vi "Quote and Escape JSON string.vi"(11 "Plain Text":string) -> (3 "<JSON>":string caption="JSON string (quoted and escaped)")   [LabVIEW 2019, in "JSONtext.lvlib"]
uses:
  JSONtext.lvlib
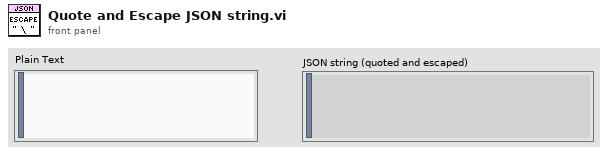
[diagram p1: front panel]
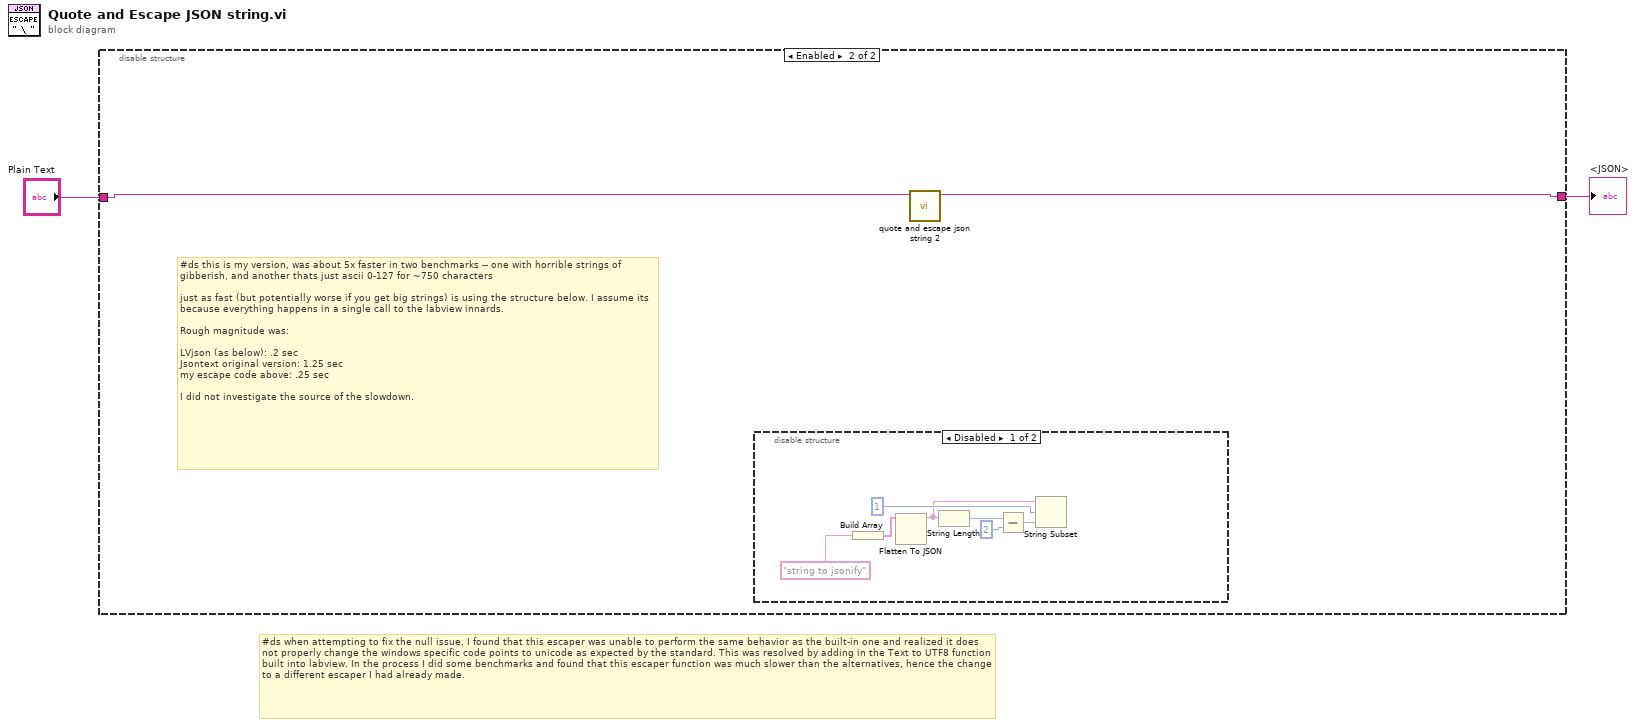
[diagram p0: block diagram]
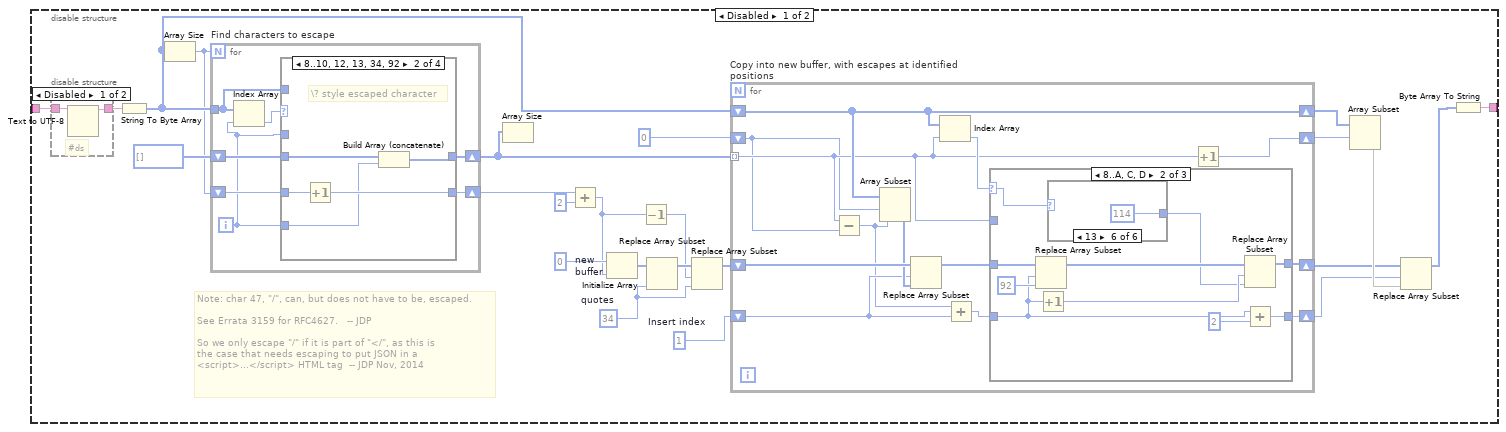
[diagram p2: hidden frame]
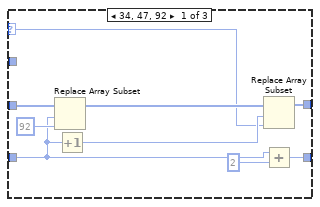
[diagram p4: hidden frame]
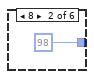
[diagram p6: hidden frame]
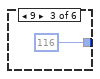
[diagram p7: hidden frame]
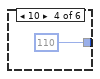
[diagram p8: hidden frame]
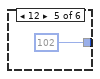
[diagram p9: hidden frame]
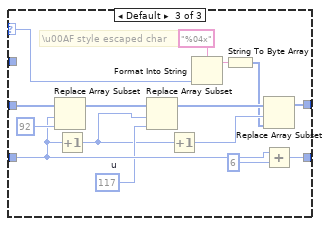
[diagram p10: hidden frame]
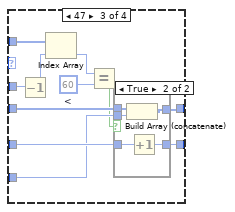
[diagram p12: hidden frame]
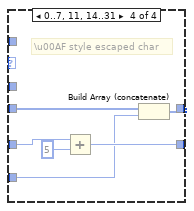
[diagram p14: hidden frame]
diagram:
  # "#ds when attempting to fix the null issue, I found that this escaper was unable to perform the same behavior as the built-in one and realized it does not properly change the windows specific code points to unicode as expected by the standard. This was resolved by adding in the Text to UTF8 function built into labview. In the process I did some benchmarks and found that this escaper function was much slower than the alternatives, hence the change to a different escaper I had already made."
  n1 = disable-structure shown="Enabled" {
    disable-tunnel: [w26 w120] -> w2
    disable-tunnel: "Plain Text" -> [w4 w121]
    frame Disabled {
      w7 = u8 34  # quotes
      w17 = 1  # Insert index
      # "Note: char 47, \"/\", can, but does not have to be, escaped.\n\nSee Errata 3159 for RFC4627.   -- JDP\n\nSo we only escape \"/\" if it is part of \"</\", as this is\nthe case that needs escaping to put JSON in a\n<script>...</script> HTML tag  -- JDP Nov, 2014"
      n2 = disable-structure shown="Disabled" {
        disable-tunnel: w4 -> [w28 w29]
        disable-tunnel: [w27 w29] -> w3
        frame Disabled {
          # "#ds"
          n3 = Text to UTF-8(11:w28) -> (3:w27:string)  [unwired: 2 in, 1 out]
        }
        frame Enabled {
        }
      }
      n4 = String To Byte Array(string=w3) -> (unsigned byte array=w21:u8[])
      n5 = Array Size(array=w21) -> (size(s)=w20:i32)
      n6 = for "Find characters to escape" {
        N: w20 -> [_]
        tunnel: w21 -> [w83]
        shift-right: [w87] -> w24
        shift-left: w20 -> [w88]
        shift-right: [w86] -> w22
        shift-left: i32[] [] -> [w85]
        i -> [w82]
        n7 = Index Array(array=w83, index=w82) -> (element=w84:u8)
        n8 = case shown="8..10, 12, 13, 34, 92" w84 {
          tunnel: w88 -> [w90 w95 w106 w116]
          tunnel: [w90 w94 w105 w119] -> w87
          tunnel: [w89 w93 w104 w118] -> w86
          tunnel: w85 -> [w89 w92 w103 w117]
          tunnel: w82 -> [_ w91 w102 w114]
          tunnel: w83 -> [_ _ w99 _]
          tunnel: w82 -> [_ _ w101 _]
          frame Default {
            # "Not escaped"
          }
          frame 8..10, 12, 13, 34, 92 {
            # "\\? style escaped character"
            n9 = Increment(x=w95) -> (x+1=w94:i32)
            n10 = Build Array (concatenate)(w92, w91) -> (w93:i32[])
          }
          frame 47 {
            w97 = u8 60  # <
            n11 = Decrement(x=w101) -> (x-1=w100:i32)
            n12 = Index Array(array=w99, index=w100) -> (element=w98:u8)
            n13 = Equal?(x=w98, y=w97) -> (x = y?=w96:bool)
            n14 = case shown="True" w96 {
              tunnel: w106 -> [w107 w113]
              tunnel: [w107 w112] -> w105
              tunnel: [w108 w111] -> w104
              tunnel: w103 -> [w108 w110]
              tunnel: w102 -> [_ w109]
              frame False {
              }
              frame True {
                n15 = Build Array (concatenate)(w110, w109) -> (w111:i32[])
                n16 = Increment(x=w113) -> (x+1=w112:i32)
              }
            }
          }
          frame 0..7, 11, 14..31 {
            # "\\u00AF style escaped char"
            n17 = Add(x=w116, y=5) -> (x+y=w119:i32)
            n18 = Build Array (concatenate)(w117, w114) -> (w118:i32[])
          }
        }
      }
      n19 = Array Size(array=w22) -> ()  [unwired: 1 out]
      n20 = Add(x=w24, y=2) -> (x+y=w9:i32)
      n21 = Initialize Array "new\nbuffer"(u8 0, w9) -> (w18:u8[])
      n22 = Decrement(x=w9) -> (x-1=w8:i32)
      n23 = Replace Array Subset(array=w18, new element=w7) -> (w11:u8[])  [unwired: 1 in]
      n24 = Replace Array Subset(array=w11, new element=w7, index=w8) -> (w10:u8[])
      n25 = for "Copy into new buffer, with escapes at identified positions" {
        tunnel: w22 -> [w32] mode=indexing
        shift-right: [w37] -> w14
        shift-left: w21 -> [w37]
        shift-right: [w36] -> w13
        shift-left: w17 -> [w35]
        shift-right: [w38] -> w15
        shift-left: w10 -> [w41]
        shift-right: [w30] -> w5
        shift-left: 0 -> [w31]
        n26 = Subtract(x=w32, y=w31) -> (x-y=w33:i32)
        n27 = Array Subset(array=w37, index=w31, length=w33) -> (w40:u8[])
        n28 = Replace Array Subset(array=w41, new element=w40, index=w35) -> (w39:u8[])
        n29 = Index Array(array=w37, index=w32) -> (element=w42:u8)
        n30 = Add(x=w33, y=w35) -> (x+y=w34:i32)
        n31 = case shown="8..A, C, D" w42 {
          selector: w42 -> [w47 w53 w73]
          tunnel: w39 -> [w51 w61 w81]
          tunnel: w32 -> [_ _ _]
          tunnel: [w46 w57 w79] -> w38
          tunnel: w34 -> [w43 w54 w76]
          tunnel: [w44 w55 w77] -> w36
          frame 34, 47, 92 {
            n32 = Replace Array Subset(array=w51, new element=u8 92 ("new element/subarray"), index=w43) -> (w49:u8[])
            n33 = Increment(x=w43) -> (x+1=w48:i32)
            n34 = Replace Array Subset(array=w49, new element=w47, index=w48) -> (w46:u8[])
            n35 = Add(x=w43, y=2) -> (x+y=w44:i32)
          }
          frame 8..10, 12, 13 {
            n36 = Replace Array Subset(array=w61, new element=u8 92 ("new element/subarray"), index=w54) -> (w59:u8[])
            n37 = Increment(x=w54) -> (x+1=w58:i32)
            n38 = case shown="13" w53 {
              tunnel: [_ u8 98 u8 116 u8 110 u8 102 u8 114] -> w52
              frame 0, Default {
              }
              frame 8 {
              }
              frame 9 {
              }
              frame 10 {
              }
              frame 12 {
              }
              frame 13 {
              }
            }
            n39 = Replace Array Subset(array=w59, new element=w52, index=w58) -> (w57:u8[])
            n40 = Add(x=w54, y=2) -> (x+y=w55:i32)
          }
          frame Default {
            w72 = u8 117  # u
            # "\\u00AF style escaped char"
            n41 = Replace Array Subset(array=w81, new element=u8 92 ("new element/subarray"), index=w76) -> (w71:u8[])
            n42 = Increment(x=w76) -> (x+1=w69:i32)
            n43 = Replace Array Subset(array=w71, new element=w72, index=w69) -> (w70:u8[])
            n44 = Increment(x=w69) -> (x+1=w68:i32)
            n45 = Format Into String(format string="%04x", w73) -> (resulting string=w74:string)  [unwired: 2 in, 1 out]
            n46 = String To Byte Array(string=w74) -> (unsigned byte array=w67:u8[])
            n47 = Replace Array Subset(array=w70, new element=w67, index=w68) -> (w79:u8[])
            n48 = Add(x=w76, y=6) -> (x+y=w77:i32)
          }
        }
        n49 = Increment(x=w32) -> (x+1=w30:i32)
      }
      n50 = Array Subset(array=w14, index=w5) -> (w16:u8[])  [unwired: 1 in]
      n51 = Replace Array Subset(array=w15, new element=w16, index=w13) -> (w23:u8[])
      n52 = Byte Array To String(unsigned byte array=w23) -> (string=w26:string)
    }
    frame Enabled {
      # "#ds this is my version, was about 5x faster in two benchmarks -- one with horrible strings of gibberish, and another thats just ascii 0-127 for ~750 characters\n\njust as fast (but potentially worse if you get big strings) is using the structure below. I assume its because everything happens in a single call to the labview innards.\n\nRough magnitude was:\n\nLVjson (as below): .2 sec\nJsontext original version: 1.25 sec\nmy escape code above: .25 sec\n\nI did not investigate the source of the slowdown."
      n53 = disable-structure shown="Disabled" {
        frame Disabled {
          n54 = Build Array("string to jsonify") -> (w127:string[])
          n55 = Flatten To JSON(anything=w127) -> (JSON string=w124:string)  [unwired: 2 in, 1 out]
          n56 = String Length(string=w124) -> (length=w125:i32)
          n57 = Subtract(x=w125, y=2 ("x")) -> (x-y=w123:i32)
          n58 = String Subset(string=w124, offset (0)=1, length (rest)=w123) -> ()  [unwired: 1 out]
        }
        frame Enabled {
        }
      }
      n59 = call "quote and escape json string 2.vi"("base string"=w121) -> ("String out"=w120:string)  [unwired: 10 in]
    }
  }
  "<JSON>" <- w2
